vi "set gain attempt 1.vi"() -> ()   [LabVIEW 2009]
panel:
  in  "Gain":dbl=50.0
  out "error out":errorcluster
  out "VISA resource name out":refnum<visa-resource-name>
  in  "error in (no error)":errorcluster
  in  "VISA resource name":refnum<visa-resource-name>="GPIB0::12::INSTR"
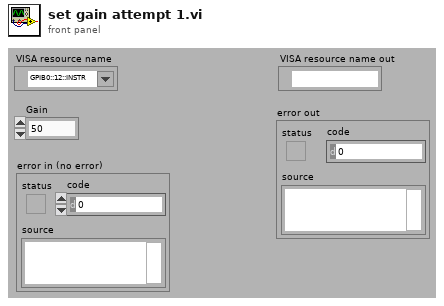
[diagram p1: front panel]
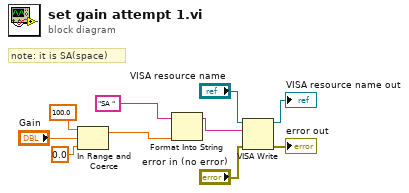
[diagram p0: block diagram]
diagram:
  # "note: it is SA(space)"
  n1 = In Range and Coerce(upper limit=100.0, x="Gain", lower limit=0.0) -> (coerced(x)=w3:dbl)  [unwired: 1 out]
  n2 = Format Into String(initial string="SA " ("write string"), w3) -> (resulting string=w1:string)  [unwired: 2 in, 1 out]
  n3 = VISA Write(VISA resource name="VISA resource name", write buffer=w1, error in (no error)="error in (no error)") -> (VISA resource name out=→"VISA resource name out":refnum<visa-resource-name>, error out=→"error out":errorcluster)  [unwired: 1 out]
